vi "Set Attribute.Instrument.vi"(8 "error in (no error)":errorcluster, 10 "Attribute.Debug":refnum<class "Attribute.Instrument.lvclass">, 11 "SMO":refnum<class "SMO.lvclass">) -> (0 "error out":errorcluster, 3 "SMO out":refnum<class "SMO.lvclass">)   [LabVIEW 2019, in "Instrument Attributes.lvlib" / "SMO.Mediator.lvclass"]
uses:
  SMO.Mediator.lvclass
  <vilib>/JKI/JKI SMO/SMO/SMO.lvclass
  Attribute.Instrument/Attribute.Instrument.lvclass
  C:/Program Files (x86)/National Instruments/LabVIEW 2019/vi.lib/JKI/JKI SMO/Support/Attribute/Attribute.lvclass
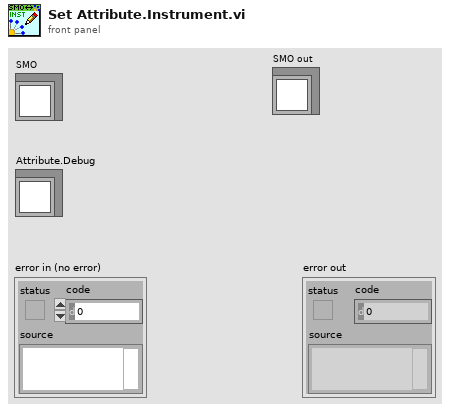
[diagram p1: front panel]
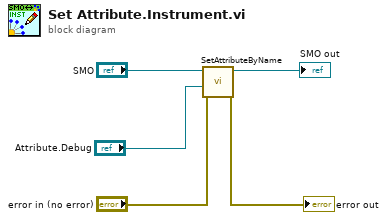
[diagram p0: block diagram]
diagram:
  n1 = call <vilib>:"SetAttributeByName.vi"("error in (no error)"="error in (no error)", "Attribute"="Attribute.Debug", "SMO in"="SMO") -> ("error out"=→"error out":errorcluster, "SMO out"=→"SMO out":refnum<class "SMO.lvclass">)  [unwired: 6 in, 1 out]
